vi "335 log(SubVI).vi"(11 "Instrument":T1={"335 Resource"="", "Input (0:A)"=0, "Instrument Type"=enum."PPMS", "quantum design"=refnum, "Heater Output (1:1)"=0, "semaphore"=refnum, "TCP master instance"=refnum, "335 Status"=refnum, "M24C Resource"="GPIB0::24::INSTR", "4G supply"="GPIB0::24::INSTR", "Temp Status 24C"=refnum, "Temp"=refnum, "9T信号"=refnum, "limit"={"Field limit"=0.0, "Field rate limit"=0.0, "Temp limit"=0.0, "Temp low limit"=0.0, "Temp rate limit "=0.0}, "4g supply status"=refnum, "vi路径"="", "325 Resource "="GPIB0::13::INSTR", "Input (0:A) 325"=0, "Input (1;B)"=1, "in-plane"="", "out-plane"="", "in-plane"=FALSE, "out-plane"=FALSE, "in plane 信号"=refnum, "pzt volt"=refnum, "Aborting"=refnum, "数据文件"=refnum, "warning"=refnum, "750 visa"="", "750 rotate"="", "335 Status 2"=refnum} {"Input (1;B)" items=["A", "B"]; "Input (0:A) 325" items=["A", "B"]; "Input (0:A)" items=["A", "B"]; "Heater Output (1:1)" items=["1"=1, "2"=2]}) -> (3 "簇":T5 {"Heater Range Loop 2" items=["Off", "Low (On)", "Medium", "High"]; "Heater Range" items=["Off", "Low (On)", "Medium", "High"]})   [LabVIEW 2019, in "Get value.lvlib"]
uses:
  Get value.lvlib
  ctl/Instrument.ctl
  <vilib>/NI/Modbus Library/API/Master/Modbus Master.lvclass
  ctl/Instrument Type.ctl
  lib/QDInstrument.dll
  ctl/335 state.ctl
  ctl/limit.ctl
  ctl/9T mag field stauts.ctl
  ctl/warning.ctl
  lib/Lake Shore 335/Lake Shore 335.lvlib
  lib/Lake Shore 325/Lake Shore 325.lvlib
panel:
  out "error out":errorcluster
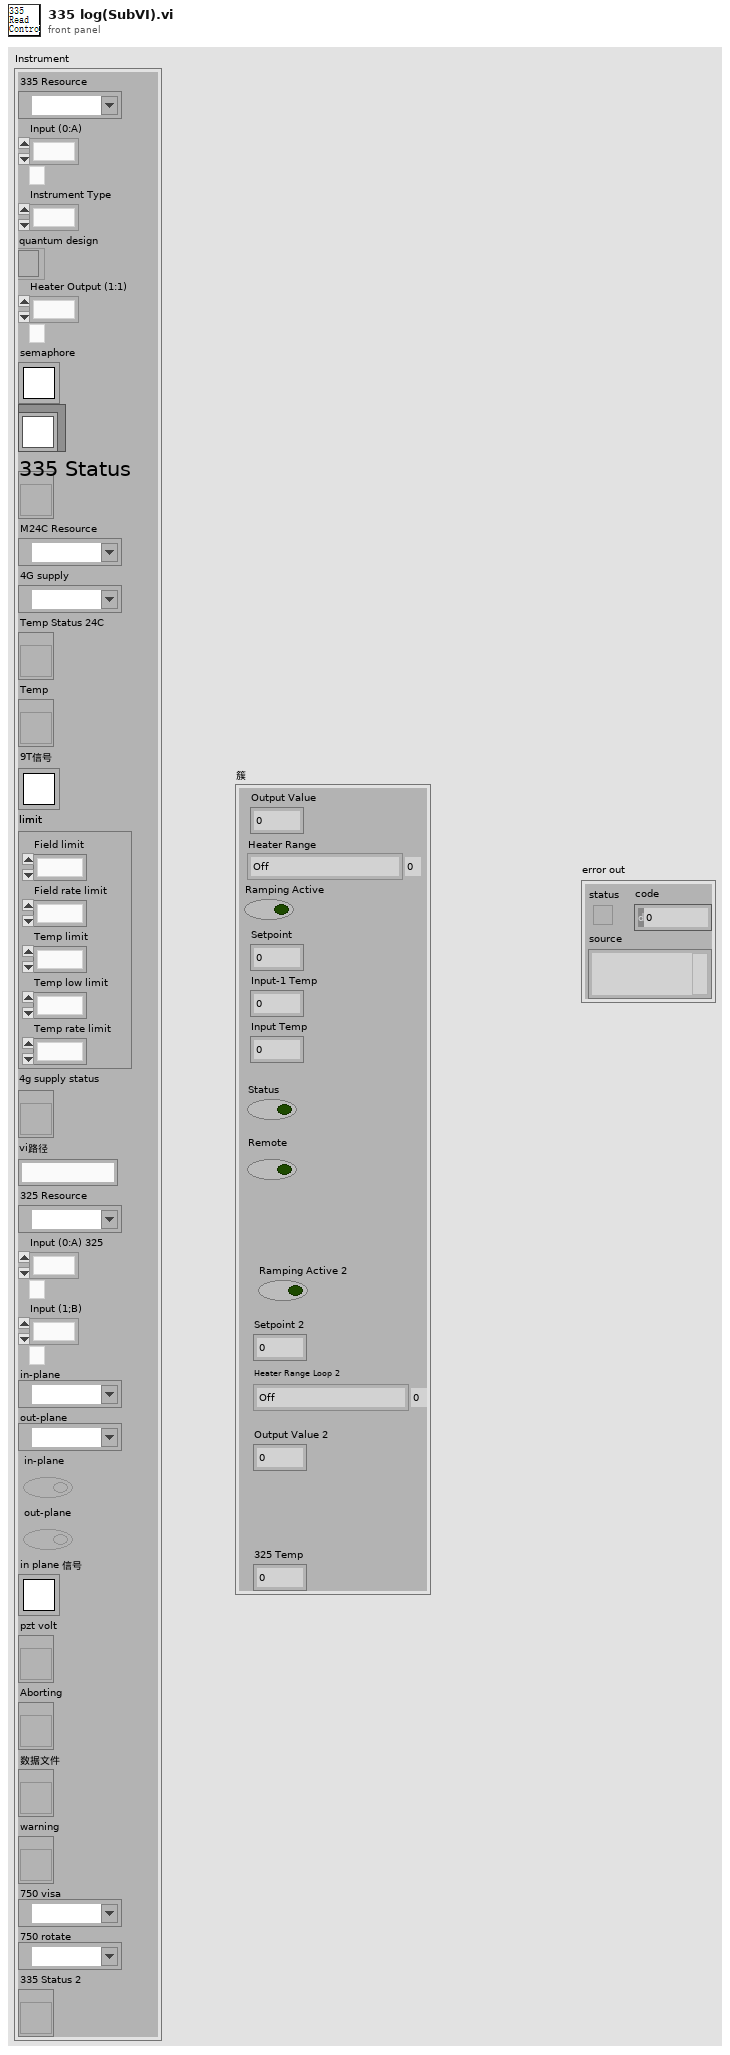
[diagram p1: front panel]
types:
  T1 = typedef "Instrument.ctl" = cluster{"335 Resource":refnum<visa-resource-name>, "Input (0:A)":u16, "Instrument Type":T2, "quantum design":refnum<k24>, "Heater Output (1:1)":u16, "semaphore":T3, "TCP master instance":refnum<class "Modbus Master.lvclass">, "335 Status":refnum<vi>, "M24C Resource":refnum<visa-resource-name>, "4G supply":refnum<visa-resource-name>, "Temp Status 24C":refnum<vi>, "Temp":refnum<vi>, "9T信号":T3, "limit":T4, "4g supply status":refnum<vi>, "vi路径":string, "325 Resource ":refnum<visa-resource-name>, "Input (0:A) 325":u16, "Input (1;B)":u16, "in-plane":refnum<visa-resource-name>, "out-plane":refnum<visa-resource-name>, "in-plane":bool, "out-plane":bool, "in plane 信号":T3, "pzt volt":refnum<vi>, "Aborting":refnum<vi>, "数据文件":refnum<vi>, "warning":refnum<vi>, "750 visa":refnum<visa-resource-name>, "750 rotate":refnum<visa-resource-name>, "335 Status 2":refnum<vi>}
  T2 = typedef "Instrument Type.ctl" = enum16{"PPMS", "VersaLab", "DynaCool", "SVSM", "PPMS-Rotate", "Lakeshore335", "lengtou2", "9T mag", "9T cmag rotate", "test"}
  T3 = typedef "Semaphore RefNum" = refnum<k1>
  T4 = typedef "limit.ctl" = cluster{"Field limit":dbl, "Field rate limit":dbl, "Temp limit":dbl, "Temp low limit":dbl, "Temp rate limit ":dbl}
  T5 = cluster{"Output Value":dbl, "Ramping Active":bool, "Setpoint":dbl, "Input-1 Temp":dbl, "Input Temp":dbl, "Status":bool, "Remote":bool, "325 Temp":dbl, "Ramping Active 2":bool, "Setpoint 2":dbl, "Output Value 2":dbl, "Heater Range ":u16, "Heater Range Loop 2":u16}
  T6 = cluster{"Output Value":dbl, "Ramping Active":bool, "Setpoint":dbl, "Sensor Data":dbl, "Sensor Data":dbl, "Boolean":bool, "Boolean":bool, "Sensor Data":dbl, "Ramping Active":bool, "Setpoint":dbl, "Output Value":dbl, "Heater Range ":u16, "Heater Range ":u16}
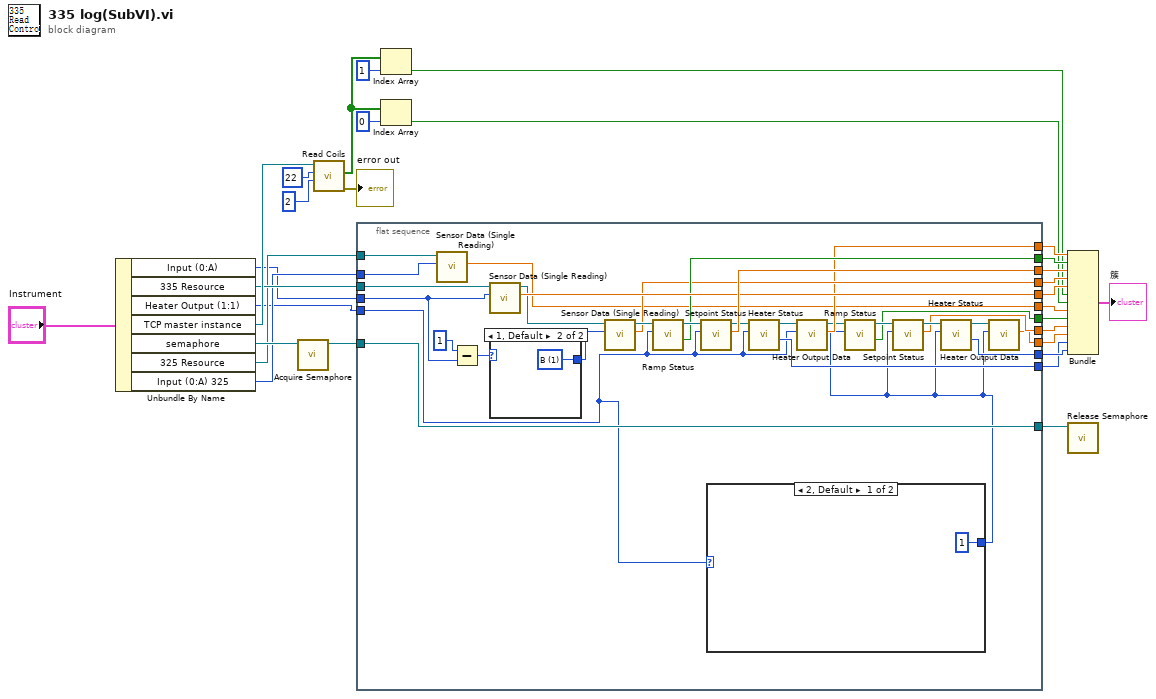
[diagram p0: block diagram]
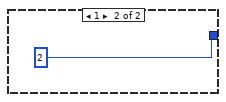
[diagram p2: hidden frame]
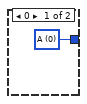
[diagram p3: hidden frame]
diagram:
  n1 = Unbundle By Name("Instrument") -> ("Input (0:A)"=w9:u16, "335 Resource"=w19:refnum<visa-resource-name>, "Heater Output (1:1)"=w1:u16, "TCP master instance"=w30:refnum<class "Modbus Master.lvclass">, "semaphore"=w18:T3, "325 Resource"=w17:refnum<visa-resource-name>, "Input (0:A) 325"=w16:u16)
  n2 = call <vilib>:"Acquire Semaphore.vi"("semaphore"=w18) -> ("semaphore out"=w22:T3)  [unwired: 4 in, 2 out]
  n3 = call-dynamic "Read Coils.vi"("number of inputs"=u16 2, "starting address"=u16 22, "Modbus master in"=w30) -> ("error out"=→"error out":errorcluster, "coils"=w29:bool[])  [unwired: 6 in, 1 out]
  n4 = flat-sequence {
    tunnel: [w60] -> w11
    tunnel: w19 -> [w58]
    tunnel: [w55] -> w8
    tunnel: w22 -> [w54]
    tunnel: [w54] -> w23
    tunnel: [w46] -> w2
    tunnel: [w47] -> w24
    tunnel: [w53] -> w12
    tunnel: w1 -> [w32]
    tunnel: w9 -> [w52]
    tunnel: [w48] -> w10
    tunnel: w17 -> [w45]
    tunnel: w16 -> [w44]
    tunnel: [w43] -> w5
    tunnel: [w38] -> w15
    tunnel: [w37] -> w14
    tunnel: [w36] -> w3
    tunnel: [w35] -> w4
    frame #0 {
      n5 = call "Sensor Data (Single Reading).vi"("Sensor Input (0:A)"=w44, "VISA resource name"=w45) -> ("Sensor Data"=w43:dbl)  [unwired: 7 in, 2 out]
      n6 = Subtract(x=u16 1, y=w52) -> (x-y=w34:u16)
      n7 = call "Sensor Data (Single Reading).vi"("Input (0:A)"=w52, "VISA resource name"=w58) -> ("Sensor Data"=w55:dbl, "VISA resource name out"=w50:refnum<visa-resource-name>)  [unwired: 7 in, 1 out]
      n8 = case shown="1, Default" w34 {
        tunnel: [w63 w64] -> w33
        frame 0 {
          w63 = u16 0 items=["A", "B"] ("Input (0:A)")
        }
        frame 1, Default {
          w64 = u16 1 items=["A", "B"] ("Input (0:A)")
        }
      }
      n9 = call "Sensor Data (Single Reading).vi"("Input (0:A)"=w33, "VISA resource name"=w50) -> ("Sensor Data"=w48:dbl, "VISA resource name out"=w49:refnum<visa-resource-name>)  [unwired: 7 in, 1 out]
      n10 = call "Ramp Status.vi"("Output's Control Loop (1:1)"=w32, "VISA resource name"=w49) -> ("Ramping Active"=w53:bool, "VISA resource name out"=w59:refnum<visa-resource-name>)  [unwired: 5 in, 3 out]
      n11 = call "Setpoint Status.vi"("Output (1:1)"=w32, "VISA resource name"=w59) -> ("Setpoint"=w60:dbl, "VISA resource name out"=w57:refnum<visa-resource-name>)  [unwired: 7 in, 1 out]
      n12 = case shown="2, Default" w32 {
        tunnel: [1 2] -> w31
        frame 2, Default {
        }
        frame 1 {
        }
      }
      n13 = call "Heater Status.vi"("Heater Output (1:1)"=w32, "VISA resource name"=w57) -> ("Heater Range"=w46:u16, "VISA resource name out"=w56:refnum<visa-resource-name>)  [unwired: 5 in, 3 out]
      n14 = call "Heater Output Data.vi"("Heater Output (1:1)"=w32, "VISA resource name"=w56) -> ("Output Value"=w47:dbl, "VISA resource name out"=w42:refnum<visa-resource-name>)  [unwired: 7 in, 1 out]
      n15 = call "Ramp Status.vi"("Output's Control Loop (1:1)"=w31, "VISA resource name"=w42) -> ("Ramping Active"=w38:bool, "VISA resource name out"=w41:refnum<visa-resource-name>)  [unwired: 5 in, 3 out]
      n16 = call "Setpoint Status.vi"("Output (1:1)"=w31, "VISA resource name"=w41) -> ("Setpoint"=w37:dbl, "VISA resource name out"=w40:refnum<visa-resource-name>)  [unwired: 7 in, 1 out]
      n17 = call "Heater Status.vi"("Heater Output (1:1)"=w31, "VISA resource name"=w40) -> ("Heater Range"=w36:u16, "VISA resource name out"=w39:refnum<visa-resource-name>)  [unwired: 5 in, 3 out]
      n18 = call "Heater Output Data.vi"("Heater Output (1:1)"=w31, "VISA resource name"=w39) -> ("Output Value"=w35:dbl)  [unwired: 7 in, 2 out]
    }
  }
  n19 = Index Array(array=w29, index=1) -> (element=w7:bool)
  n20 = Index Array(array=w29, index=0) -> (element=w6:bool)
  n21 = Bundle("Output Value"=w24, "Ramping Active"=w12, "Setpoint"=w11, "Sensor Data"=w10, "Sensor Data"=w8, "Boolean"=w7, "Boolean"=w6, "Sensor Data"=w5, "Ramping Active"=w15, "Setpoint"=w14, "Output Value"=w4, "Heater Range"=w2, "Heater Range"=w3) -> (→"簇":T6)  [unwired: 1 in]
  n22 = call <vilib>:"Release Semaphore.vi"("semaphore"=w23) -> ()  [unwired: 5 in, 2 out]
